vi "UTILITY Simple PID.vi"(6 "K(0.1)":dbl=0.3, 8 "Error In":errorcluster, 9 "GPM Target(3)":dbl, 10 "GPM reading":dbl, 11 "Previous MicroAmp":dbl) -> (0 "Error Out":errorcluster, 2 "Adjustment Factor":dbl, 3 "New MicroAmp":dbl)   [LabVIEW 2019]
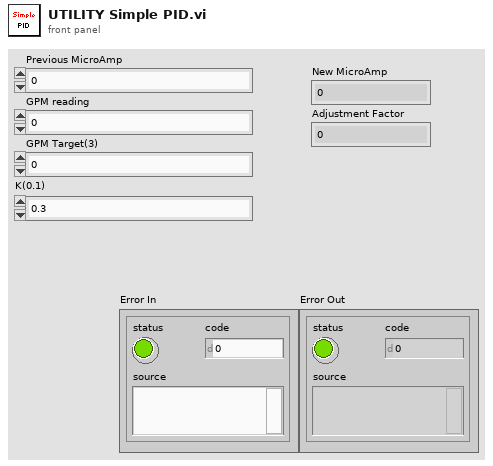
[diagram p1: front panel]
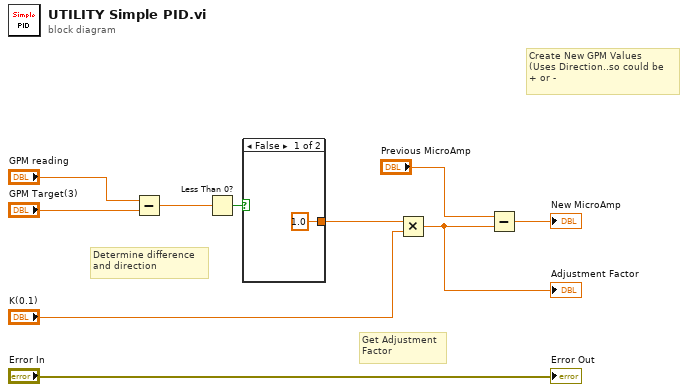
[diagram p0: block diagram]
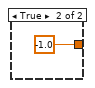
[diagram p2: hidden frame]
diagram:
  # "Create New GPM Values\n(Uses Direction..so could be \n+ or -"
  # "Get Adjustment\nFactor"
  # "Determine difference \nand direction"
  n1 = Subtract(x="GPM reading", y="GPM Target(3)") -> (x-y=w3:dbl)
  n2 = Less Than 0?(x=w3) -> (x < 0?=w1:bool)
  n3 = case shown="False" w1 {
    tunnel: [1.0 -1.0] -> w2
    frame False {
    }
    frame True {
    }
  }
  n4 = Multiply(x=w2, y="K(0.1)") -> (x*y=w6:dbl)
  "Adjustment Factor" <- w6
  n5 = Subtract(x="Previous MicroAmp", y=w6) -> (x-y=→"New MicroAmp":dbl)
  "Error Out" <- "Error In"
